vi "CLD 4 Event Structure Time Out Front Panel.vi"() -> ()   [LabVIEW 2014]
doc: "CLD-Übung 4"
uses:
  CLD 3/CLD3 Timer Mode.ctl
panel:
  in  "Dekrementieren":bool
  out "Fehler (Ausgang)":T1
  in  "Fehler (Eingang)":T1
  out "Zeit ist verstrichen":bool
  out "Zählwert":string="0"
  in  "Inkrementieren":bool
  in  "VI anhalten":bool
  in  "Zielzeit (s)":dbl=2.0
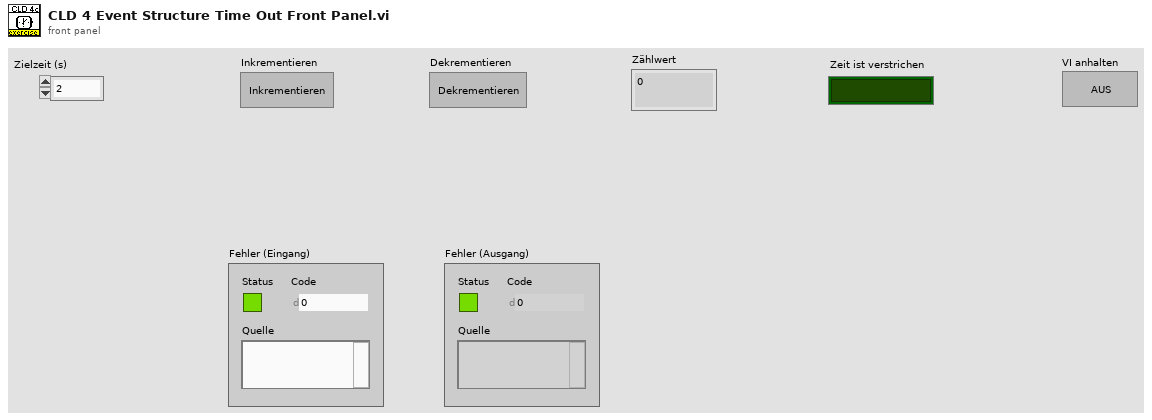
[diagram p1: front panel]
types:
  T1 = cluster{"Status":bool, "Code":i32, "Quelle":string}
  T2 = typedef "CLD3 Timer Mode.ctl" = enum16{"Zurücksetzen", "Verstrichen"}
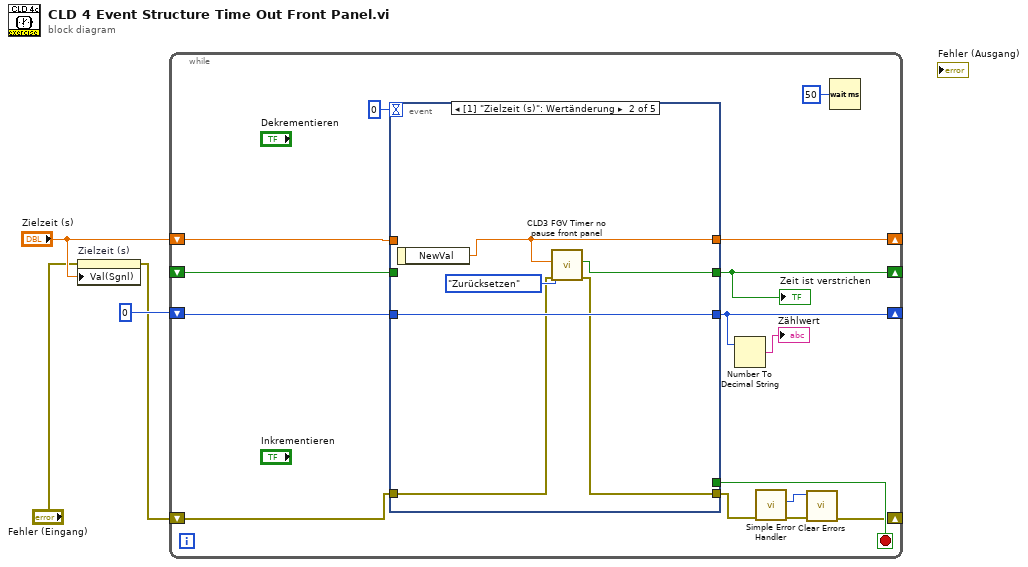
[diagram p0: block diagram]
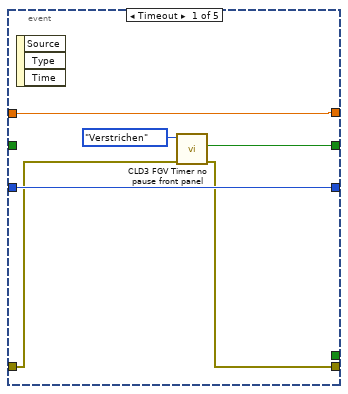
[diagram p2: hidden frame]
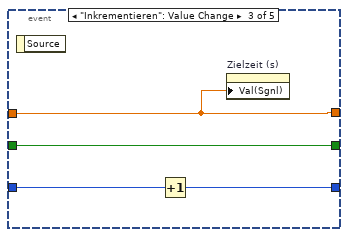
[diagram p3: hidden frame]
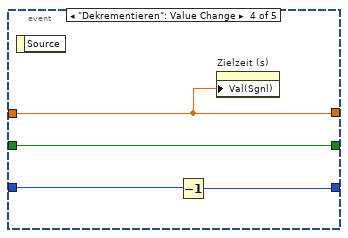
[diagram p4: hidden frame]
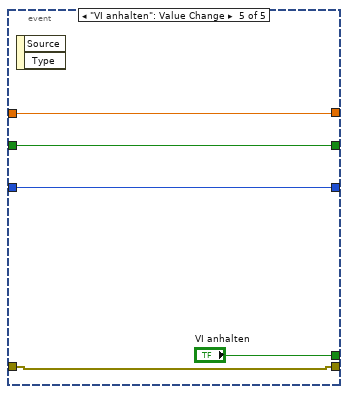
[diagram p5: hidden frame]
diagram:
  n1 = property on="Zielzeit (s)" class="DigWert (strikt)"(error in="Fehler (Eingang)", "Val(Sgnl)"="Zielzeit (s)") -> (error out=w1:errorcluster)  [unwired: 1 in, 1 out]
  n2 = while {
    shift-right: [w14] -> _
    shift-left: u32 0 -> [w16]
    shift-right: [w12] -> _
    shift-left: "Zielzeit (s)" -> [w13]
    shift-right: [w11] -> _
    shift-left: _ -> [w10]
    shift-right: [w5] -> _
    shift-left: w1 -> [w9]
    stop <- w17 stop-if-true
    n3 = event shown="[1] \"Zielzeit (s)\": Wertänderung" {
      selector: _ -> [_ _ _ _ _]
      dyn-events: _ -> [_ _ _ _ _]
      timeout: 0 -> [_ _ _ _ _]
      tunnel: [_ _ _ _ "VI anhalten"] -> w17
      tunnel: w16 -> [w25 w29 w35 w39 w43]
      tunnel: [w25 w29 w34 w38 w43] -> w14
      tunnel: w13 -> [w23 _ w32 w36 w42]
      tunnel: [w23 w31 w32 w36 w42] -> w12
      tunnel: [w22 w28 w33 w37 w41] -> w11
      tunnel: w10 -> [_ _ w33 w37 w41]
      tunnel: w9 -> [w21 w27 _ _ w40]
      tunnel: [w20 w26 _ _ w40] -> w8
      event Timeout {
        n4 = event-data() -> ()  [unwired: 1 in, 3 out]
        n5 = call "CLD3 FGV Timer no pause front panel.vi"("Fehler (Eingang, kein Fehler)"=w21, "Timer-Task"=CLD3_Timer_Mode."Verstrichen") -> ("Fehler (Ausgang)"=w20:errorcluster, "Verstrichene Zeit?"=w22:bool)  [unwired: 7 in, 1 out]
      }
      event "Zielzeit (s)": Value Change {
        n6 = event-data() -> ("NewVal"=w31:dbl)  [unwired: 1 in]
        n7 = call "CLD3 FGV Timer no pause front panel.vi"("Fehler (Eingang, kein Fehler)"=w27, "Warten"=w31, "Timer-Task"=CLD3_Timer_Mode."Zurücksetzen") -> ("Fehler (Ausgang)"=w26:errorcluster, "Verstrichene Zeit?"=w28:bool)  [unwired: 6 in, 1 out]
      }
      event "Inkrementieren": Value Change {
        n8 = event-data() -> ()  [unwired: 1 in, 1 out]
        n9 = Increment(x=w35) -> (x+1=w34:u32)
        n10 = property on="Zielzeit (s)" class="DigWert (strikt)"("Val(Sgnl)"=w32) -> ()  [unwired: 2 in, 2 out]
      }
      event "Dekrementieren": Value Change {
        n11 = event-data() -> ()  [unwired: 1 in, 1 out]
        n12 = Decrement(x=w39) -> (x-1=w38:u32)
        n13 = property on="Zielzeit (s)" class="DigWert (strikt)"("Val(Sgnl)"=w36) -> ()  [unwired: 2 in, 2 out]
      }
      event "VI anhalten": Value Change {
        n14 = event-data() -> ()  [unwired: 1 in, 2 out]
      }
    }
    "Zeit ist verstrichen" <- w11
    n15 = Number To Decimal String(number=w14) -> (decimal integer string=→"Zählwert":string)  [unwired: 1 in]
    n16 = call <vilib>:"Simple Error Handler.vi"("error in (no error)"=w8) -> ("code out"=w6:i32, "error out"=w7:errorcluster)  [unwired: 4 in, 3 out]
    n17 = call <vilib>:"Clear Errors.vi"("error in (no error)"=w7, "specific error code to clear (0: all)"=w6) -> ("error out"=w5:errorcluster)  [unwired: 4 in, 1 out]
    n18 = Wait (ms)(milliseconds to wait=u32 50 ("Zu wartende ms")) -> ()  [unwired: 1 out]
  }
